vi "read_attributes.vi"(8 "error in (no error)":errorcluster, 11 "RandomForestClassifier in":refnum<class "RandomForestClassifier.lvclass">) -> (0 "error out":errorcluster, 2 "attributes":T1, 3 "RandomForestClassifier out":refnum<class "RandomForestClassifier.lvclass">)   [LabVIEW 2020, in "RandomForestClassifier.lvclass"]
uses:
  RandomForestClassifier.lvclass
  Controls/random_forest_classifier_attributes.ctl
  RandomForestClassifier.lvclass/RandomForestClassifier.ctl
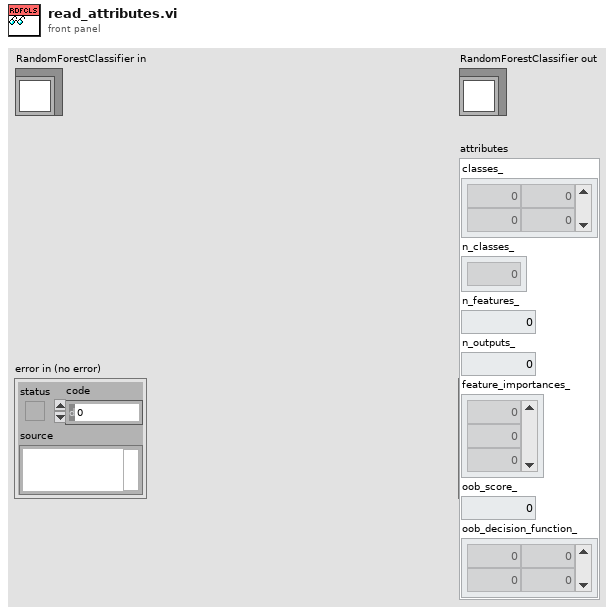
[diagram p1: front panel]
types:
  T1 = typedef "random_forest_classifier_attributes.ctl" = cluster{"classes_":dbl[][], "n_classes_":dbl[], "n_features_":dbl, "n_outputs_":dbl, "feature_importances_":dbl[], "oob_score_":dbl, "oob_decision_function_":dbl[][]}
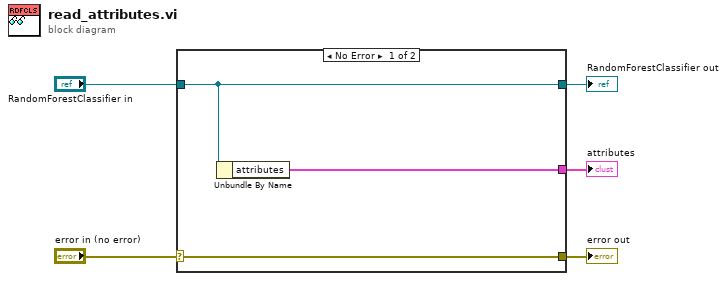
[diagram p0: block diagram]
diagram:
  n1 = case shown="No Error" "error in (no error)" {
    selector: "error in (no error)" -> [w8 w9]
    tunnel: [w8 w9] -> w4
    tunnel: [w7 w10] -> w2
    tunnel: "RandomForestClassifier in" -> [w7 w10]
    tunnel: [w6 _] -> w1
    frame No Error {
      n2 = Unbundle By Name(w7) -> ("attributes"=w6:T1)
    }
    frame Error {
    }
  }
  "error out" <- w4
  "RandomForestClassifier out" <- w2
  "attributes" <- w1
